vi "Compute controls(SubVI).vi"(8 "error in (no error)":errorcluster, 11 "Array of Joint Positions in":dbl[][](array[numeric])) -> (0 "error out":errorcluster, 3 "Control Cluster out":T1={"Roll"=0.09503769, "Pitch"=0.11711881, "Vertical Speed"=0.0, "Yaw Speed"=-0.05722916} {"Yaw Speed" scale=-1.0..1.0; "Vertical Speed" scale=-1.0..1.0; "Pitch" scale=-1.0..1.0; "Roll" scale=-1.0..1.0})   [LabVIEW 2014]
uses:
  Resources/Others/Control cluster.ctl
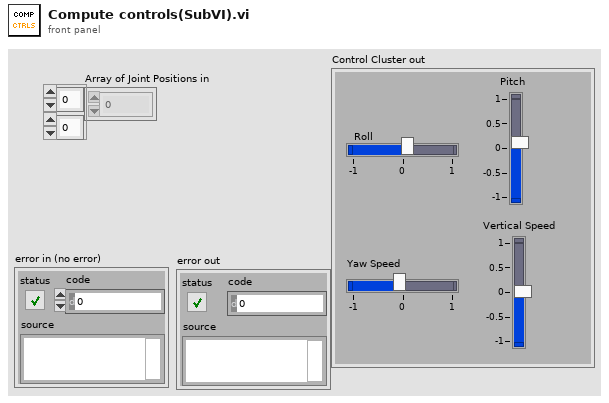
[diagram p1: front panel]
types:
  T1 = typedef "Control cluster.ctl" = cluster{"Roll":sgl, "Pitch":sgl, "Vertical Speed":sgl, "Yaw Speed":sgl}
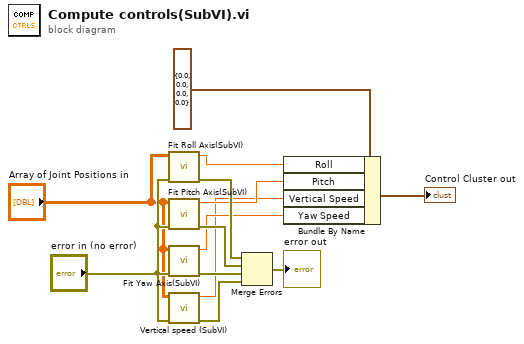
[diagram p0: block diagram]
diagram:
  n1 = call "Fit Roll Axis(SubVI).vi"("error in (no error)"="error in (no error)", "Array of Joint Positions in"="Array of Joint Positions in") -> ("error out"=w7:errorcluster, "Roll"=w4:dbl)  [unwired: 8 in]
  n2 = call "Fit Pitch Axis(SubVI).vi"("error in (no error)"="error in (no error)", "Array of Joint Positions in"="Array of Joint Positions in") -> ("error out"=w8:errorcluster, "Pitch"=w3:dbl)  [unwired: 8 in]
  n3 = call "Fit Yaw Axis(SubVI).vi"("error in (no error)"="error in (no error)", "Array of Joint Positions in in"="Array of Joint Positions in") -> ("error out"=w9:errorcluster, "Yaw"=w2:dbl)  [unwired: 8 in]
  n4 = call "Vertical speed (SubVI).vi"("error in (no error)"="error in (no error)", "Array of Joint Positions in"="Array of Joint Positions in") -> ("error out"=w13:errorcluster, "Vertical Speed"=w1:dbl)  [unwired: 7 in, 1 out]
  n5 = Merge Errors(w7, w8, w9, w13) -> (→"error out":errorcluster)
  n6 = Bundle By Name(cluster=T1 {"Roll"=0.0, "Pitch"=0.0, "Vertical Speed"=0.0, "Yaw Speed"=0.0} ("Control Cluster out 2"), "Roll"=w4, "Pitch"=w3, "Vertical Speed"=w1, "Yaw Speed"=w2) -> (→"Control Cluster out":T1)
